vi "Map Tags to Channels.vi"(7 "instance id":string, 8 "error in (no error)":errorcluster, 9 "String Array":string[][](array[string]), 10 "channels":refnum<class "TBM channel.lvclass">[](array[class]), 11 "engine configuration in":refnum<class "engine configuration.lvclass">) -> (0 "error out":errorcluster, 3 "engine configuration out":refnum<class "engine configuration.lvclass">)   [LabVIEW 2015, in "Modbus Module editor node.lvclass"]
uses:
  Modbus Module editor node.lvclass
  <vilib>/NI/Module Execution Interface/Engine Configuration/engine configuration.lvclass
  <vilib>/NI/Tag Bus Module Framework/channel/TBM channel.lvclass
  <vilib>/NI/Tag Bus/tag/tag descriptor.lvclass/tag descriptor.ctl
  <vilib>/NI/Tag Bus/tag/tag descriptor.lvclass
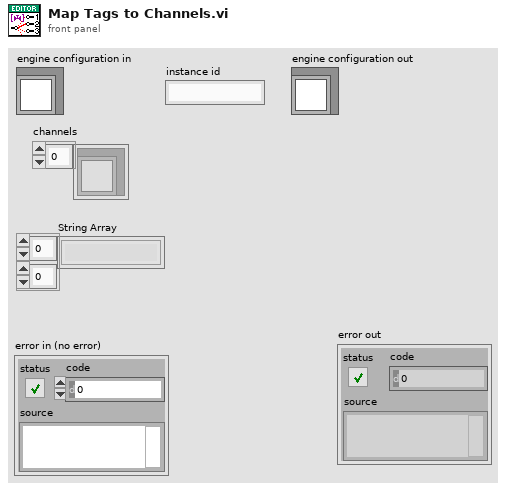
[diagram p1: front panel]
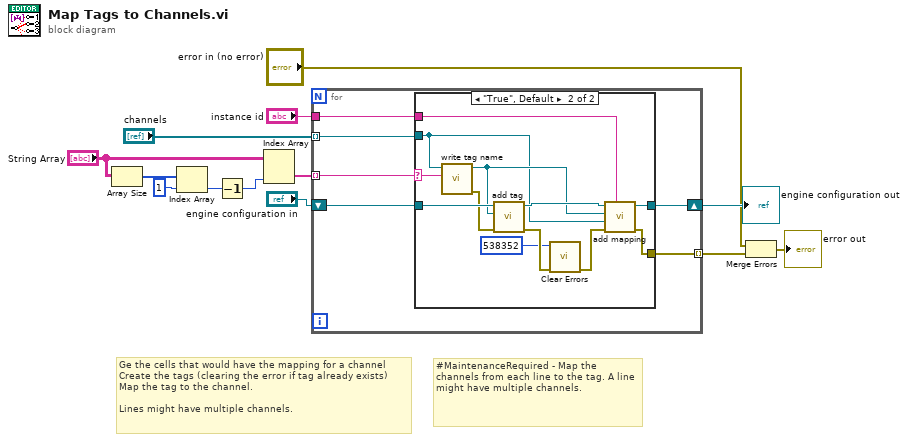
[diagram p0: block diagram]
diagram:
  # "#MaintenanceRequired - Map the channels from each line to the tag. A line might have multiple channels."
  # "Ge the cells that would have the mapping for a channel\nCreate the tags (clearing the error if tag already exists) \nMap the tag to the channel.\n\nLines might have multiple channels."
  n1 = Array Size(array="String Array") -> (size(s)=w9:i32[])
  n2 = Index Array(array=w9, index=1) -> (element=w7:i32)
  n3 = Decrement(x=w7) -> (x-1=w6:i32)
  n4 = Index Array(array="String Array", index (col)=w6) -> (element=w4:string[])  [unwired: 1 in]
  n5 = for {
    tunnel: "channels" -> [w15] mode=indexing
    tunnel: w4 -> [w14] mode=indexing
    shift-right: [w19] -> w11
    shift-left: "engine configuration in" -> [w16]
    tunnel: "instance id" -> [w18]
    tunnel: [w17] -> w13 mode=indexing
    n6 = case shown="\"True\", Default" w14 {
      selector: w14 -> [_ w21]
      tunnel: [w20 w32] -> w19
      tunnel: w18 -> [_ w31]
      tunnel: [_ w30] -> w17
      tunnel: w16 -> [w20 w29]
      tunnel: w15 -> [_ w26]
      frame "" {
      }
      frame "True", Default {
        n7 = call <vilib>:"write tag name.vi"("name"=w21, "system tag in"=w26) -> ("error out"=w25:errorcluster, "system tag out"=w27:refnum<class "TBM channel.lvclass">)  [unwired: 8 in]
        n8 = call-dynamic "add tag.vi"("error in"=w25, "tag descriptor"=w27, "engine configuration in"=w29) -> ("error out"=w24:errorcluster, "engine configuration out"=w28:refnum<class "engine configuration.lvclass">)  [unwired: 7 in]
        n9 = call <vilib>:"Clear Errors.vi"("error in (no error)"=w24, "specific error code to clear (0: all)"=538352) -> ("error out"=w23:errorcluster)  [unwired: 4 in, 1 out]
        n10 = call-dynamic "add mapping.vi"("owner ID"=w31, "error in"=w23, "channel"=w26, "tag descriptor"=w27, "engine configuration"=w28) -> ("error out"=w30:errorcluster, "engine configuration out"=w32:refnum<class "engine configuration.lvclass">)  [unwired: 5 in]
      }
    }
  }
  "engine configuration out" <- w11
  n11 = Merge Errors("error in (no error)", w13) -> (→"error out":errorcluster)
